vi "DB - Get Keys.vi"(7 "subVI":bool=TRUE, 8 "error in (no error)":errorcluster, 10 "DB.Schema.Table":string="MyDB1.ck.orders", 11 "Refnum in":T3) -> (0 "error out":errorcluster, 1 "Foreign Keys":string[](array[string])=["OrderNo"], 2 "Primary Key":string[](array[string])=["OrderNo"], 3 "Refnum out":T3)   [LabVIEW 2013]
uses:
  <vilib>/addons/database/Connection.llb/Conn ObjectReference.ctl
  Controls/DB - DB.Schema.Table.ctl
  <vilib>/addons/database/Connection.llb/Conn Execute.vi
  <vilib>/addons/database/Recordset.llb/Rec Fetch Recordset Data (R).vi
  <vilib>/addons/database/Recordset.llb/Rec Destroy - Connection.vi
  <vilib>/addons/database/Connection.llb/DB Tools Open Connec (String).vi
  <vilib>/addons/database/_DB Variant To Data/Database Variant To Data.xnode
  <vilib>/addons/database/NI_Database_API.lvlib
panel:
  out "DB.Schema.Table":T1
  out "SQL Query 1":string
  out "SQL Query":string
  out "call chain":string[](array[string])
  in  "Connection Information":T2={"Connection "="SQL Server 32bit HPEnvy", "Username"="admin", "Password"="admin123"}
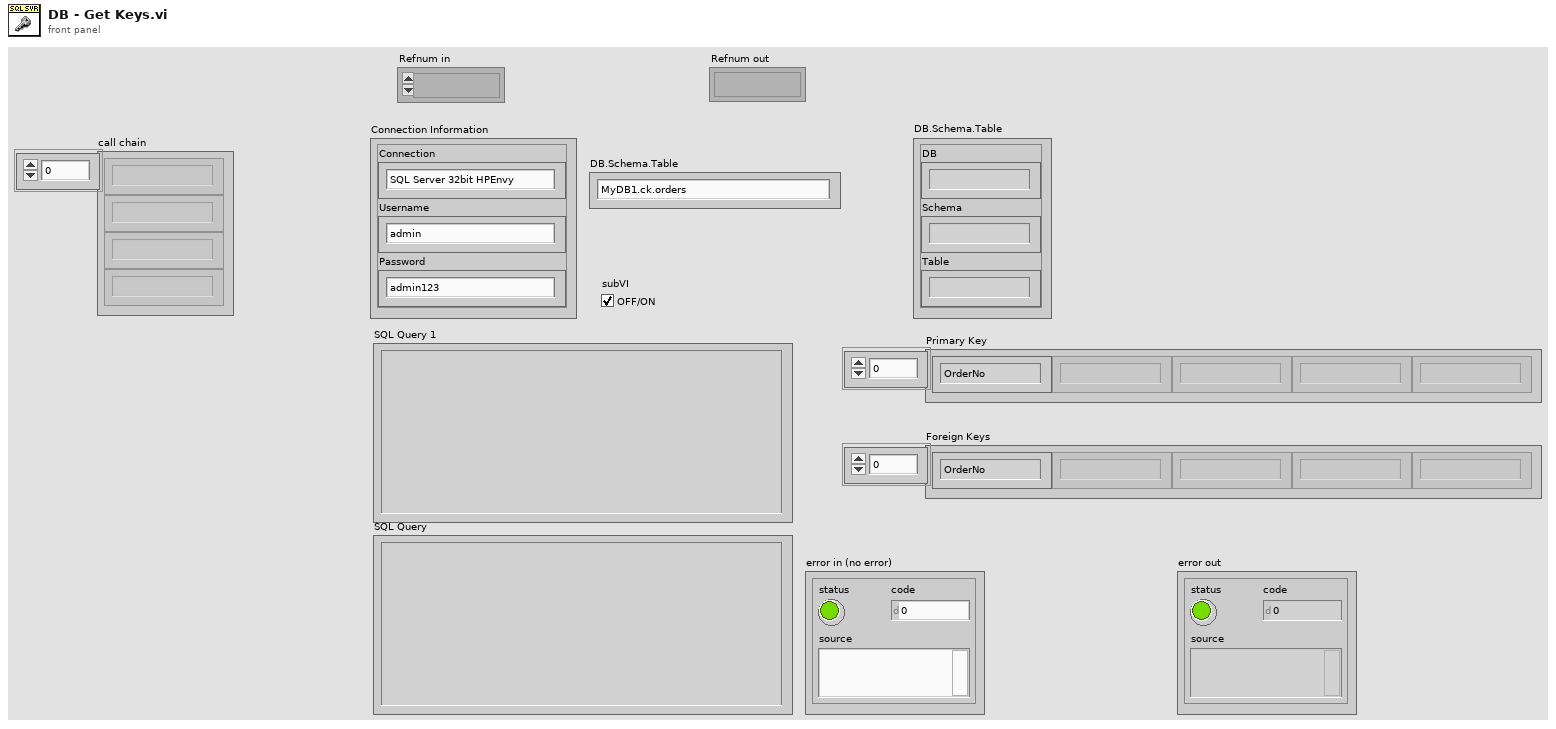
[diagram p1: front panel]
types:
  T1 = typedef "DB - DB.Schema.Table.ctl" = cluster{"DB":string, "Schema":string, "Table":string}
  T2 = cluster{"Connection ":string, "Username":string, "Password":string}
  T3 = typedef "NI_Database_API.lvlib/Conn ObjectReference.ctl" = refnum<k1>
  T4 = typedef "NI_Database_API.lvlib/Rec ObjectReference.ctl" = refnum<k1>
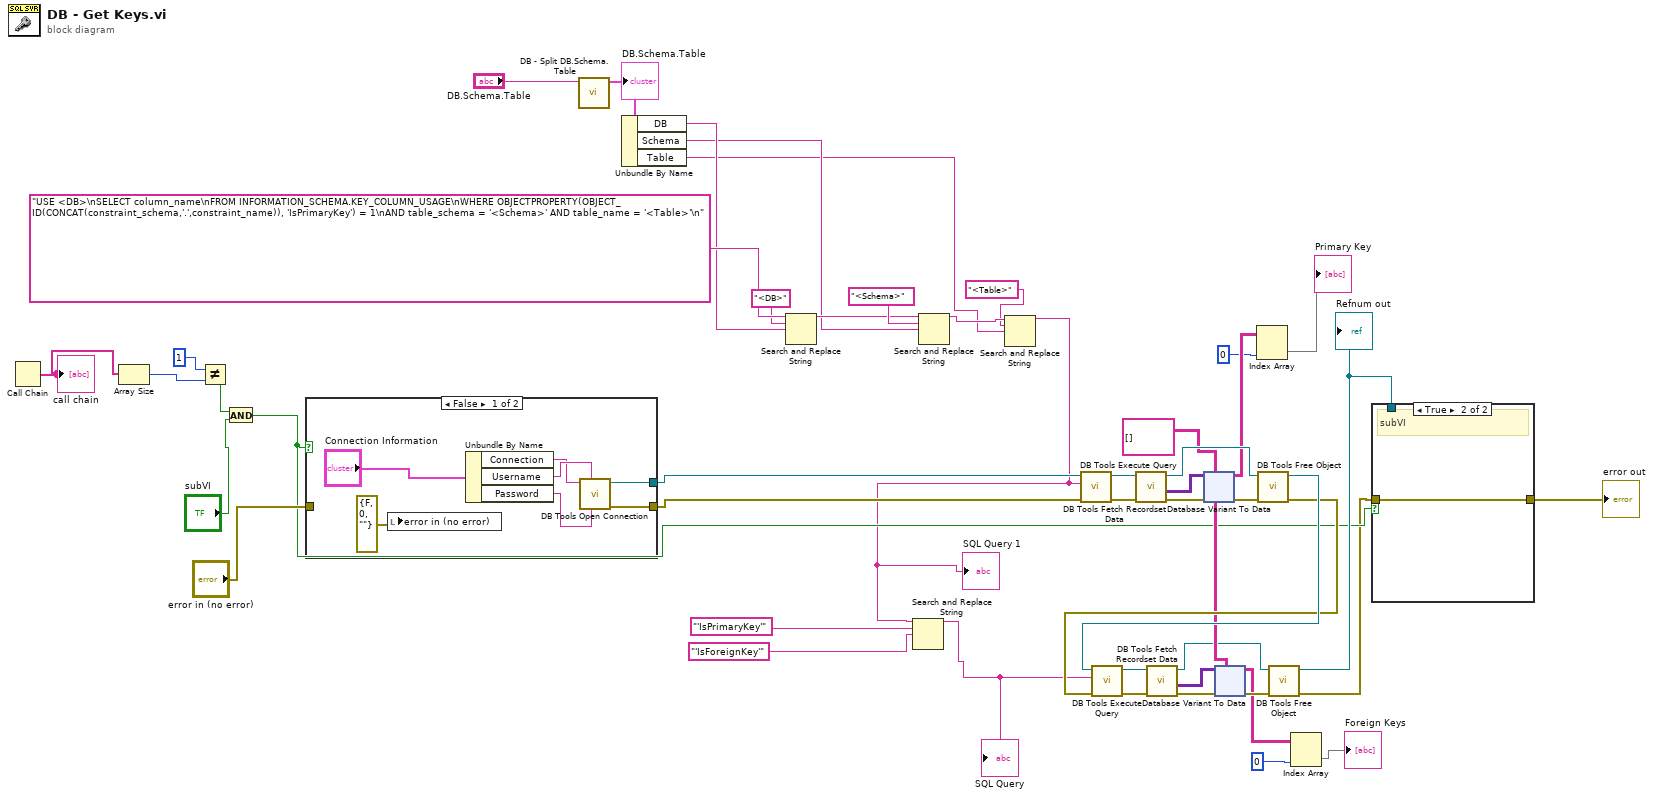
[diagram p0: block diagram]
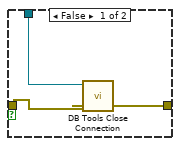
[diagram p2: hidden frame]
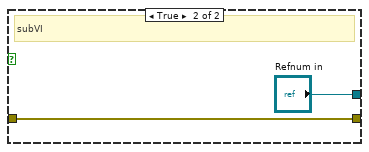
[diagram p3: hidden frame]
diagram:
  w28 = string[][] []
  n1 = Call Chain() -> (call chain=w20:string[])
  "call chain" <- w20
  n2 = Array Size(array=w20) -> (size(s)=w19:i32)
  n3 = Not Equal?(x=1, y=w19) -> (x != y?=w18:bool)
  n4 = And(x=w18, y="subVI") -> (x .and. y?=w15:bool)
  n5 = case shown="False" w15 {
    tunnel: [w51 "Refnum in"] -> w40
    tunnel: "error in (no error)" -> [_ w56]
    tunnel: [w50 w56] -> w41
    frame False {
      n6 = local write "error in (no error)"(errorcluster {"status"=FALSE, "code"=0, "source"=""} ("error constant")) -> ()
      n7 = Unbundle By Name("Connection Information") -> ("Connection"=w53:string, "Username"=w54:string, "Password"=w52:string)
      n8 = call-poly <vilib>:"DB Tools Open Connection.vi"("password"=w52, "userID"=w54, "connection information"=w53) -> ("error out"=w50:errorcluster, "connection reference"=w51:T3)  [unwired: 5 in]
    }
    frame True {
      # "subVI"
    }
  }
  n9 = call "DB - Split DB.Schema.Table.vi"("DB.Schema.Table"="DB.Schema.Table") -> ("DB.Schema.Table"=w5:T1)  [unwired: 10 in]
  "DB.Schema.Table" <- w5
  n10 = Unbundle By Name(w5) -> ("DB"=w4:string, "Schema"=w3:string, "Table"=w2:string)
  n11 = Search and Replace String(input string="USE <DB>\nSELECT column_name\nFROM INFORMATION_SCHEMA.KEY_COLUMN_USAGE\nWHERE OBJECTPROPERTY(OBJECT_ID(CONCAT(constraint_schema,'.',constraint_name)), 'IsPrimaryKey') = 1\nAND table_schema = '<Schema>' AND table_name = '<Table>'\n" ("string"), search string="<DB>", replace string=w4) -> (result string=w8:string)  [unwired: 5 in, 3 out]
  n12 = Search and Replace String(input string=w8, search string="<Schema>", replace string=w3) -> (result string=w11:string)  [unwired: 5 in, 3 out]
  n13 = Search and Replace String(input string=w11, search string="<Table>", replace string=w2) -> (result string=w10:string)  [unwired: 5 in, 3 out]
  "SQL Query 1" <- w10
  n14 = Search and Replace String(input string=w10, search string="'IsPrimaryKey'", replace string="'IsForeignKey'") -> (result string=w14:string)  [unwired: 5 in, 3 out]
  "SQL Query" <- w14
  n15 = call-poly <vilib>:"DB Tools Execute Query.vi"("error in (no error)"=w41, "SQL query"=w10, "connection reference"=w40) -> ("error out"=w45:errorcluster, "recordset reference"=w43:T4)  [unwired: 5 in]
  n16 = call-poly <vilib>:"DB Tools Fetch Recordset Data.vi"("error in (no error)"=w45, "recordset reference"=w43) -> ("error out"=w47:errorcluster, "recordset data"=w46:variant[][], "recordset reference out"=w44:T4)  [unwired: 3 in]
  n17 = xnode "Database Variant To Data"("database variant"=w46, "error in (no error)"=w47, "type"=w28) -> ("data"=w38:string[][], "error out"=w48:errorcluster)
  n18 = Index Array(array=w38, index (col)=0) -> (element=→"Primary Key":string[])  [unwired: 1 in]
  n19 = call-poly <vilib>:"DB Tools Free Object.vi"("error in (no error)"=w48, "recordset reference"=w44) -> ("error out"=w29:errorcluster, "connection reference"=w30:T3)  [unwired: 8 in]
  n20 = call-poly <vilib>:"DB Tools Execute Query.vi"("error in (no error)"=w29, "SQL query"=w14, "connection reference"=w30) -> ("error out"=w34:errorcluster, "recordset reference"=w35:T4)  [unwired: 5 in]
  n21 = call-poly <vilib>:"DB Tools Fetch Recordset Data.vi"("error in (no error)"=w34, "recordset reference"=w35) -> ("error out"=w32:errorcluster, "recordset data"=w33:variant[][], "recordset reference out"=w24:T4)  [unwired: 3 in]
  n22 = xnode "Database Variant To Data"("database variant"=w33, "error in (no error)"=w32, "type"=w28) -> ("data"=w26:string[][], "error out"=w31:errorcluster)
  n23 = call-poly <vilib>:"DB Tools Free Object.vi"("error in (no error)"=w31, "recordset reference"=w24) -> ("error out"=w1:errorcluster, "connection reference"=w23:T3)  [unwired: 8 in]
  "Refnum out" <- w23
  n24 = Index Array(array=w26, index (col)=0) -> (element=→"Foreign Keys":string[])  [unwired: 1 in]
  n25 = case shown="True" w15 {
    tunnel: w23 -> [w60 _]
    tunnel: w1 -> [w59 w61]
    tunnel: [w58 w61] -> w39
    frame False {
      n26 = call <vilib>:"DB Tools Close Connection.vi"("error in (no error)"=w59, "connection reference"=w60) -> ("error out"=w58:errorcluster)  [unwired: 5 in]
    }
    frame True {
      # "subVI"
    }
  }
  "error out" <- w39
